vi "oa_OrderResolution to BlockSize.vi"(1 "Order resolution (order)":dbl=0.1 min=0.0, 2 "Max order to analyze":dbl=64.0 format="%.2f") -> (0 "Block size":i32)   [LabVIEW 2017]
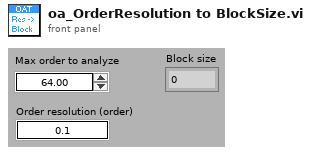
[diagram p1: front panel]
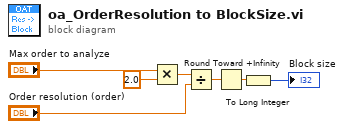
[diagram p0: block diagram]
diagram:
  n1 = Multiply(x="Max order to analyze", y=2.0) -> (x*y=w5:dbl)
  n2 = Divide(x=w5, y="Order resolution (order)") -> (x/y=w3:dbl)
  n3 = Round Toward +Infinity(x=w3) -> (ceil(x): smallest int >= x=w2:dbl)
  n4 = To Long Integer(number=w2) -> (32bit integer=→"Block size":i32)
